vi "Teleop.vi"(10 "Match Info":T2={"Autonomous Elapsed Seconds"=0.0, "TeleOp Elapsed Seconds"=0.0, "Disabled Elapsed Seconds"=0.0, "Visited Autonomous"=FALSE, "Visited TeleOp"=FALSE, "Visited Disabled"=FALSE, "Autonomous Settings"={"Autonomous Style"=enum."Independent", "VI Refnum"=refnum}}, 11 "Call Context":T3) -> ()   [LabVIEW 2015]
doc: "This VI is called for each TeleOp packet received from the DS where the robot is not disabled. It is often used to read from the joysticks and update I/O or to update setpoints for timed control loops. It should complete and return within 20 milliseconds or it may miss DS packets."
uses:
  <vilib>/Rock Robotics/WPI/DriverStation/WPI_DriverStationDerivedRobotMode.ctl
  <vilib>/Rock Robotics/WPI/DriverStation/WPI_DriverStationMatch Info.ctl
  <vilib>/Rock Robotics/WPI/Utilities/WPI_GetSetVariantRefNum.vi
  <vilib>/Rock Robotics/Network Tables/SD Write Boolean Array.vi
  <vilib>/Rock Robotics/Network Tables/SD Read Boolean.vi
  <vilib>/Rock Robotics/Network Tables/SD Read Number.vi
  Robot Global Data.vi
  <vilib>/addons/control/pid/pid.llb/PID (DBL).vi
  <vilib>/Rock Robotics/WPI/RobotDrive/WPI_RobotDriveMecanumDrive_Cartesian.vi
  <vilib>/addons/control/pid/NI_PID_pid.lvlib
panel:
  in  "UseGyro?":bool
  out "Gyro":T1(graph)
  out "Rotation Input":dbl(graph)
  out "Sample Slider 0":dbl(slide) scale=0.0..5.0
  out "Sample Boolean 1":bool
  out "Sample Boolean 0":bool
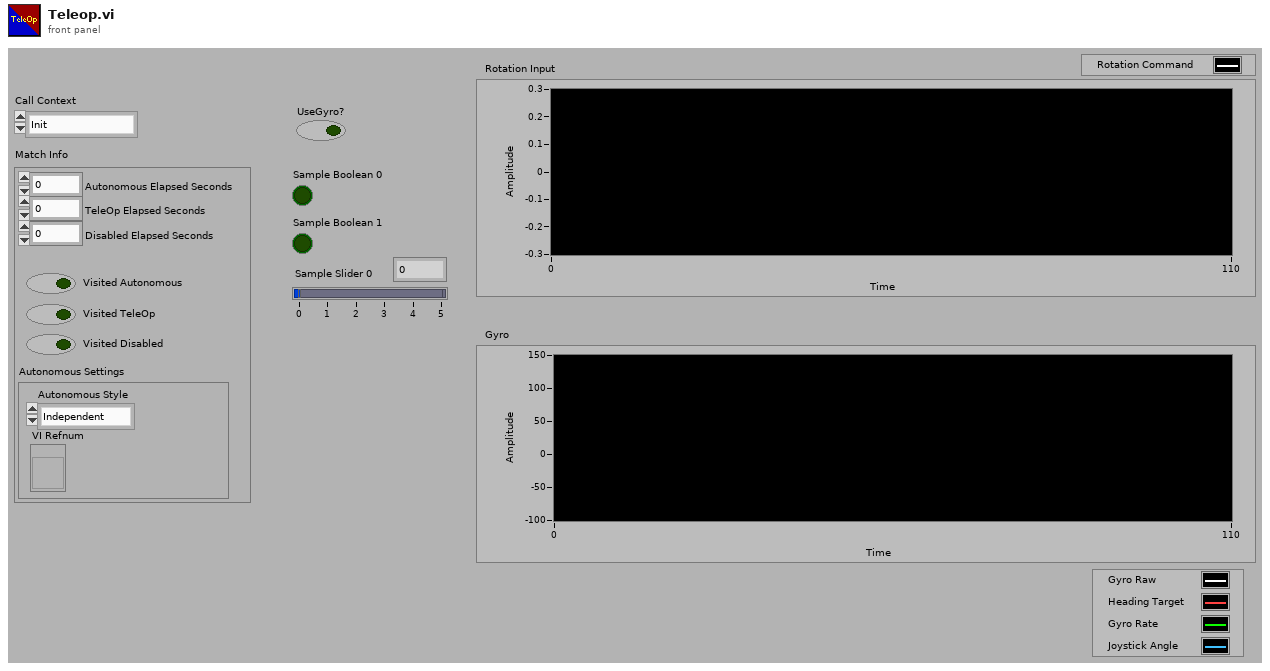
[diagram p1: front panel]
types:
  T1 = cluster{"Angle":dbl, "Heading":dbl, "Angular Rate":dbl, dbl}
  T2 = typedef "WPI_DriverStationMatch Info.ctl" = cluster{"Autonomous Elapsed Seconds":dbl, "TeleOp Elapsed Seconds":dbl, "Disabled Elapsed Seconds":dbl, "Visited Autonomous":bool, "Visited TeleOp":bool, "Visited Disabled":bool, "Autonomous Settings":cluster{"Autonomous Style":enum16{"Iterative", "Independent"}, "VI Refnum":refnum<vi>}}
  T3 = typedef "WPI_DriverStationDerivedRobotMode.ctl" = enum16{"Init", "Execute", "Stop"}
  T4 = cluster{"proportional gain (Kc)":dbl, "integral time (Ti, min)":dbl, "derivative time (Td, min)":dbl}
  T5 = typedef "WPI_JoystickDevRef.ctl" = cluster{"Device":T6}
  T6 = typedef "WPI_JoystickDeviceEnum.ctl" = enum16{"USB 0", "USB 1", "USB 2", "USB 3", "USB 4", "USB 5"}
  T7 = cluster{"Axes[0]":dbl, "Axes[1]":dbl, "Axes[2]":dbl, "Axes[3]":dbl, "Axes[4]":dbl, "Axes[5]":dbl, "Axes[6]":dbl, "Axes[7]":dbl, "Axes[8]":dbl}
  T8 = cluster{"Buttons[0]":bool, "Buttons[1]":bool, "Buttons[2]":bool, "Buttons[3]":bool, "Buttons[4]":bool, "Buttons[5]":bool, "Buttons[6]":bool, "Buttons[7]":bool, "Buttons[8]":bool}
  T9 = enum16{"CW_Fast", "CW_Slow", "CCW_Fast", "CCW_Slow", "Straight", "WaitingForStraight", "Rotate_Move"}
  T10 = cluster{"GyroHeading":dbl, "Heading":dbl, "GyroRate":dbl, dbl}
  T11 = typedef "WPI_RobotDriveDevRef.ctl" = cluster{"DevStatus":errorcluster, "Motors[]":T12[], "Square Inputs":bool, "Max Output":dbl}
  T12 = typedef "WPI_MotorControlDeviceRef.ctl" = cluster{"DeviceStatus":errorcluster, "Type":T13, "PWM":cluster{"PWM Channel":T14, "DeadBand":T15}, "CAN":cluster{"Device Number":u8, "Control Mode":T16, "Semaphore":T17, "Max Vout":dbl, "TalonSRX Control Mode":T18}, "Invert":bool}
  T13 = typedef "WPI_MotorControlType.ctl" = enum16{"PWM", "CAN", "CANTalonSRX"}
  T14 = typedef "FPGA_DIOPWMChannel.ctl" = enum8{"PWM 0", "PWM 1", "PWM 2", "PWM 3", "PWM 4", "PWM 5", "PWM 6", "PWM 7", "PWM 8", "PWM 9", "PWM MXP 0", "PWM MXP 1", "PWM MXP 2", "PWM MXP 3", "PWM MXP 4", "PWM MXP 5", "PWM MXP 6", "PWM MXP 7", "PWM MXP 8", "PWM MXP 9", "Invalid"}
  T15 = typedef "WPI_PWMDeadband.ctl" = cluster{"Name":string, "maxPositivePwm":i32, "minPositivePwm":i32, "centerPwm":i32, "maxNegativePwm":i32, "minNegativePwm":i32, "angularRange":u16}
  T16 = typedef "WPI_CANJaguar_ControlMode.ctl" = enum8{"Percent VBus", "Current", "Speed", "Position", "Voltage"}
  T17 = typedef "Semaphore RefNum" = refnum<k1>
  T18 = typedef "WPI_CANTalonSRX_APIControlMode.ctl" = enum8{"Percent VBus", "Speed", "Position", "Slave", "Unchanged / Invalid", "Voltage Compensation", "Current"}
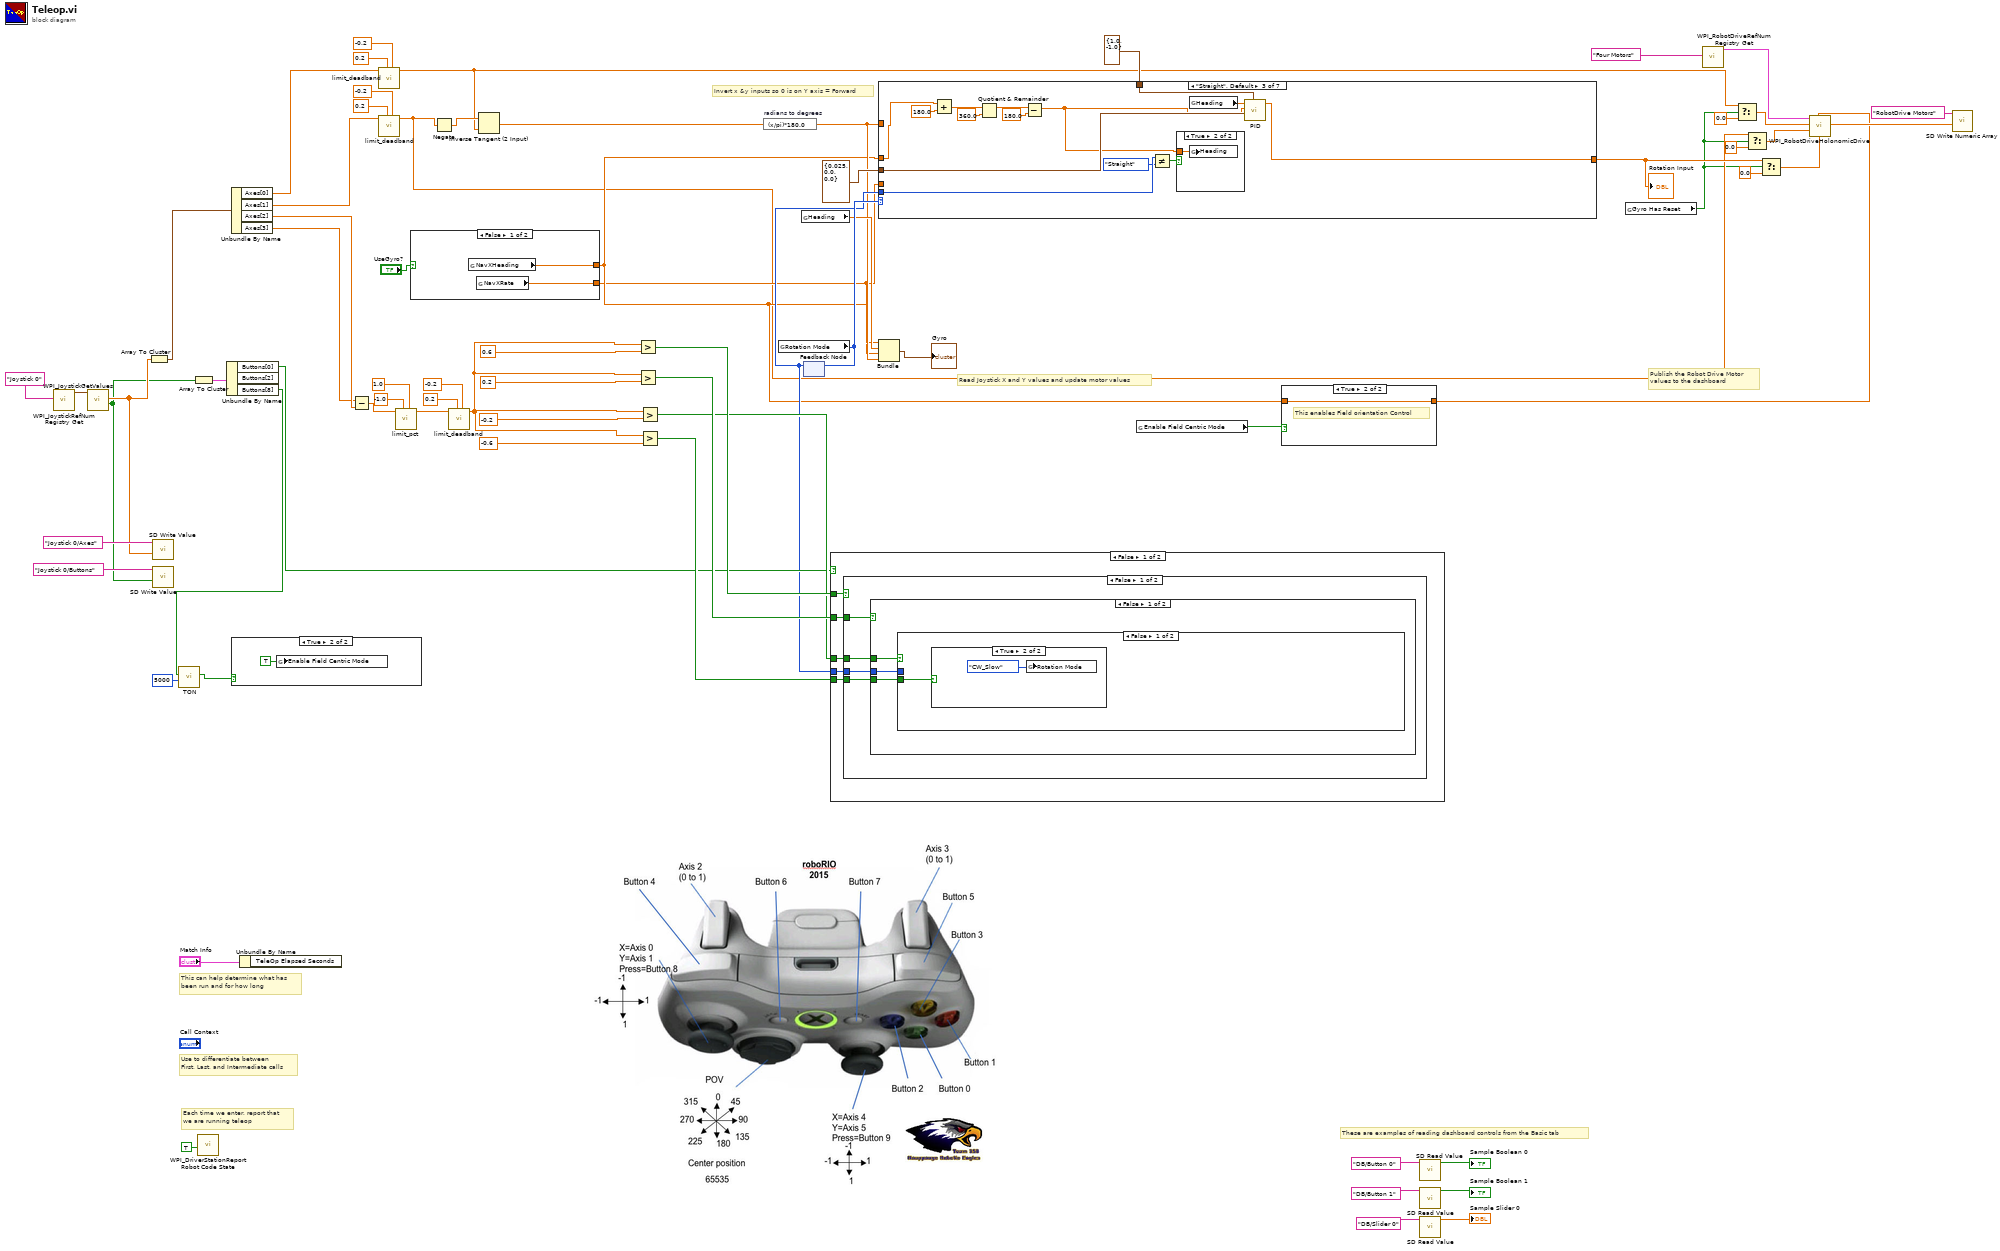
[diagram p0: block diagram]
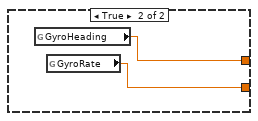
[diagram p2: hidden frame]
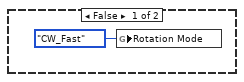
[diagram p4: hidden frame]
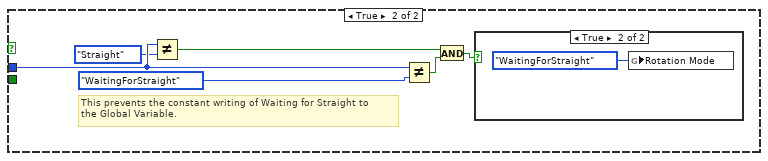
[diagram p5: hidden frame]
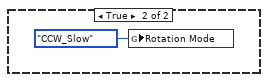
[diagram p7: hidden frame]
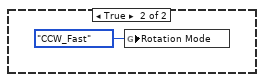
[diagram p8: hidden frame]
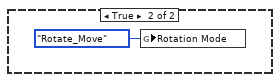
[diagram p9: hidden frame]
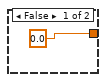
[diagram p10: hidden frame]
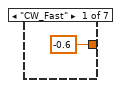
[diagram p11: hidden frame]
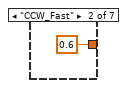
[diagram p12: hidden frame]
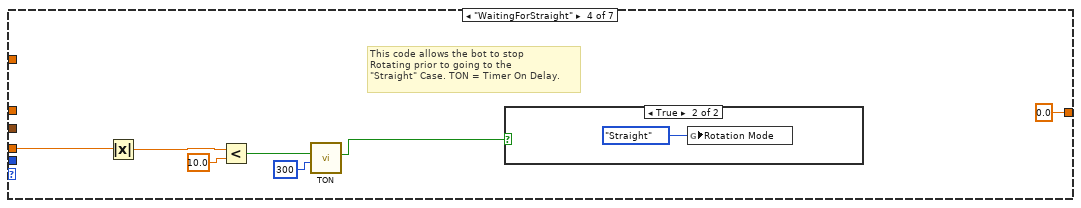
[diagram p14: hidden frame]
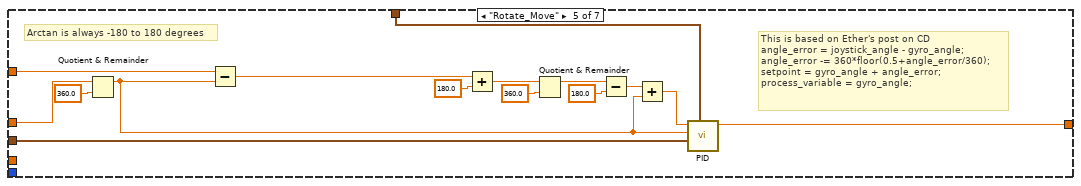
[diagram p16: hidden frame]
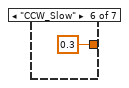
[diagram p17: hidden frame]
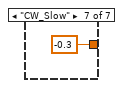
[diagram p18: hidden frame]
diagram:
  # "Invert x &y inputs so 0 is on Y axis = Forward"
  # "Publish the Robot Drive Motor\nvalues to the dashboard"
  # "Read Joystick X and Y values and update motor values"
  # "These are examples of reading dashboard controls from the Basic tab"
  # "Each time we enter, report that\nwe are running teleop"
  # "Use to differentiate between\nFirst, Last, and Intermediate calls"
  # "This can help determine what has\nbeen run and for how long"
  n1 = call <vilib>:"WPI_JoystickRefNum Registry Get.vi"("refnum name"="Joystick 0") -> ("JoystickDevRef"=w69:T5)  [unwired: 1 in, 9 out]
  n2 = call <vilib>:"WPI_JoystickGetValues.vi"("JoystickDevRef"=w69) -> ("Buttons"=w18:bool[], "Axes"=w20:dbl[])  [unwired: 6 in, 3 out]
  n3 = Array To Cluster(array=w20) -> (cluster=w19:T7)
  n4 = call-poly <vilib>:"SD Write Value.vi"("Numeric Array"=w20, "Name"="Joystick 0/Axes") -> ()  [unwired: 8 in, 2 out]
  n5 = call-poly <vilib>:"SD Write Value.vi"("Boolean Array"=w18, "Name"="Joystick 0/Buttons") -> ()  [unwired: 8 in, 2 out]
  n6 = Array To Cluster(array=w18) -> (cluster=w17:T8)
  n7 = call <vilib>:"WPI_DriverStationReport Robot Code State.vi"("TeleOp"=TRUE ("Autonomous")) -> ()  [unwired: 10 in, 1 out]
  n8 = Unbundle By Name(w17) -> ("Buttons[0]"=w36:bool, "Buttons[8]"=w12:bool)  [unwired: 1 out]
  n9 = call "TON.vi"("Delay (ms)"=u32 5000, "Input"=w12) -> ("Output"=w13:bool)  [unwired: 9 in]
  n10 = Unbundle By Name(w19) -> ("Axes[0]"=w35:dbl, "Axes[1]"=w24:dbl, "Axes[2]"=w27:dbl, "Axes[3]"=w26:dbl)
  n11 = case shown="True" w13 {
    frame False {
    }
    frame True {
      n12 = global write "Robot Global Data.vi" "Enable Field Centric Mode"(TRUE ("Enable Field Centric Mode")) -> ()
    }
  }
  n13 = Unbundle By Name("Match Info") -> ()  [unwired: 1 out]
  n14 = Subtract(x=w26, y=w27) -> (x-y=w28:dbl)
  n15 = call "limit_deadband.vi"("lower limit"=-0.2, "upper limit"=0.2, "Val"=w35) -> ("Val Out"=w3:dbl)  [unwired: 8 in]
  n16 = call "limit_deadband.vi"("lower limit"=-0.2, "upper limit"=0.2, "Val"=w24) -> ("Val Out"=w5:dbl)  [unwired: 8 in]
  n17 = call "limit_pct.vi"("upper limit"=1.0, "lower limit"=-1.0, "PCT"=w28) -> ("PCT Out"=w47:dbl)  [unwired: 8 in]
  n18 = case shown="False" "UseGyro?" {
    tunnel: [w74 w76] -> w15
    tunnel: [w73 w75] -> w14
    frame False {
      n19 = global read "Robot Global Data.vi" "NavXHeading"() -> (w74:dbl)
      n20 = global read "Robot Global Data.vi" "NavXRate"() -> (w73:dbl)
    }
    frame True {
      n21 = global read "Robot Global Data.vi" "GyroHeading"() -> (w76:dbl)
      n22 = global read "Robot Global Data.vi" "GyroRate"() -> (w75:dbl)
    }
  }
  n23 = Negate(x=w5) -> (-x=w23:dbl)
  n24 = call "limit_deadband.vi"("lower limit"=-0.2, "upper limit"=0.2, "Val"=w47) -> ("Val Out"=w40:dbl)  [unwired: 8 in]
  n25 = Inverse Tangent (2 Input)(1:w3, 2:w23) -> (0:w21:dbl)
  n26 = Greater?(x=w40, y=0.6 ("x")) -> (0:w46:bool)
  n27 = Greater?(x=w40, y=0.2 ("x")) -> (0:w45:bool)
  n28 = Greater?(x=w40, y=-0.2) -> (0:w41:bool)
  n29 = Greater?(x=w40, y=-0.6) -> (0:w38:bool)
  n30 = expression code="(x/pi)*180.0" "radians to degrees"(w21) -> (w22:dbl)
  n31 = global read "Robot Global Data.vi" "Rotation Mode"() -> (w32:T9)
  n32 = global read "Robot Global Data.vi" "Heading"() -> (w31:dbl)
  n33 = feedback #1() -> (w30:T9)  [unwired: 1 in]
  n34 = feedback-in #1(w32) -> ()
  n35 = case shown="False" w36 {
    tunnel: w46 -> [w81 _]
    tunnel: w45 -> [w80 _]
    tunnel: w41 -> [w79 _]
    tunnel: w38 -> [w78 _]
    tunnel: w30 -> [w77 _]
    frame False {
      n36 = case shown="False" w81 {
        tunnel: w80 -> [w85 _]
        tunnel: w79 -> [w84 _]
        tunnel: w78 -> [w83 _]
        tunnel: w77 -> [w82 _]
        frame False {
          n37 = case shown="False" w85 {
            tunnel: w84 -> [w88 _]
            tunnel: w83 -> [w87 _]
            tunnel: w82 -> [w86 _]
            frame False {
              n38 = case shown="False" w88 {
                tunnel: w87 -> [w89 _]
                tunnel: w86 -> [_ w97]
                frame False {
                  n39 = case shown="True" w89 {
                    frame False {
                      n40 = global write "Robot Global Data.vi" "Rotation Mode"(T9."CW_Fast" ("Rotation Mode")) -> ()
                    }
                    frame True {
                      n41 = global write "Robot Global Data.vi" "Rotation Mode"(T9."CW_Slow" ("Rotation Mode")) -> ()
                    }
                  }
                }
                frame True {
                  # "This prevents the constant writing of Waiting for Straight to \nthe Global Variable."
                  n42 = Not Equal?(x=w97, y=T9."Straight") -> (x != y?=w93:bool)
                  n43 = Not Equal?(x=w97, y=T9."WaitingForStraight") -> (x != y?=w92:bool)
                  n44 = And(x=w93, y=w92) -> (x .and. y?=w94:bool)
                  n45 = case shown="True" w94 {
                    frame False {
                    }
                    frame True {
                      n46 = global write "Robot Global Data.vi" "Rotation Mode"(T9."WaitingForStraight" ("Rotation Mode")) -> ()
                    }
                  }
                }
              }
            }
            frame True {
              n47 = global write "Robot Global Data.vi" "Rotation Mode"(T9."CCW_Slow" ("Rotation Mode")) -> ()
            }
          }
        }
        frame True {
          n48 = global write "Robot Global Data.vi" "Rotation Mode"(T9."CCW_Fast" ("Rotation Mode")) -> ()
        }
      }
    }
    frame True {
      n49 = global write "Robot Global Data.vi" "Rotation Mode"(T9."Rotate_Move" ("Rotation Mode")) -> ()
    }
  }
  n50 = case shown="\"Straight\", Default" w32 {
    tunnel: [-0.6 ("Rotation") 0.6 ("Rotation") w111 0.0 ("Rotation") w141 0.3 ("Rotation") -0.3 ("Rotation")] -> w9
    tunnel: w15 -> [_ _ w105 _ w128 _ _]
    tunnel: w14 -> [_ _ _ w120 _ _ _]
    tunnel: T4 {"proportional gain (Kc)"=0.025, "integral time (Ti, min)"=0.0, "derivative time (Td, min)"=0.0} ("PID gains") -> [_ _ w112 _ w140 _ _]
    tunnel: w22 -> [_ _ _ _ w134 _ _]
    tunnel: cluster{"output high":dbl, "output low":dbl} {"output high"=1.0, "output low"=-1.0} ("output range") -> [_ _ w113 _ w137 _ _]
    tunnel: w30 -> [_ _ w117 _ _ _ _]
    frame "CW_Fast" {
    }
    frame "CCW_Fast" {
    }
    frame "Straight", Default {
      n51 = Add(x=w105, y=180.0) -> (x+y=w108:dbl)
      n52 = Quotient & Remainder(x=w108, y=360.0) -> (x-y*floor(x/y)=w107:dbl)  [unwired: 1 out]
      n53 = Subtract(x=w107, y=180.0) -> (x-y=w104:dbl)
      n54 = Not Equal?(x=w117, y=T9."Straight" ("Rotation Mode")) -> (x != y?=w114:bool)
      n55 = case shown="True" w114 {
        tunnel: w104 -> [_ w118]
        frame False {
        }
        frame True {
          n56 = global write "Robot Global Data.vi" "Heading"(w118) -> ()
        }
      }
      n57 = global read "Robot Global Data.vi" "Heading"() -> (w115:dbl)
      n58 = call-poly <vilib>:"PID.vi"("output range"=w113, "PID gains"=w112, "process variable"=w104, "setpoint"=w115) -> ("output"=w111:dbl)  [unwired: 6 in, 1 out]
    }
    frame "WaitingForStraight" {
      # "This code allows the bot to stop \nRotating prior to going to the \n\"Straight\" Case. TON = Timer On Delay."
      n59 = Absolute Value(x=w120) -> (abs(x)=w119:dbl)
      n60 = Less?(x=w119, y=10.0) -> (x < y?=w122:bool)
      n61 = call "TON.vi"("Delay (ms)"=u32 300, "Input"=w122) -> ("Output"=w123:bool)  [unwired: 9 in]
      n62 = case shown="True" w123 {
        frame False {
        }
        frame True {
          n63 = global write "Robot Global Data.vi" "Rotation Mode"(T9."Straight" ("Rotation Mode")) -> ()
        }
      }
    }
    frame "Rotate_Move" {
      # "Arctan is always -180 to 180 degrees"
      # "This is based on Ether's post on CD\nangle_error = joystick_angle - gyro_angle;\nangle_error -= 360*floor(0.5+angle_error/360);\nsetpoint = gyro_angle + angle_error;\nprocess_variable = gyro_angle;"
      n64 = Quotient & Remainder(x=w128, y=360.0) -> (x-y*floor(x/y)=w127:dbl)  [unwired: 1 out]
      n65 = Subtract(x=w134, y=w127) -> (x-y=w136:dbl)
      n66 = Add(x=w136, y=180.0) -> (x+y=w133:dbl)
      n67 = Quotient & Remainder(x=w133, y=360.0) -> (x-y*floor(x/y)=w132:dbl)  [unwired: 1 out]
      n68 = Subtract(x=w132, y=180.0) -> (x-y=w130:dbl)
      n69 = Add(x=w130, y=w127) -> (x+y=w129:dbl)
      n70 = call-poly <vilib>:"PID.vi"("output range"=w137, "PID gains"=w140, "process variable"=w127, "setpoint"=w129) -> ("output"=w141:dbl)  [unwired: 6 in, 1 out]
    }
    frame "CCW_Slow" {
    }
    frame "CW_Slow" {
    }
  }
  "Rotation Input" <- w9
  n71 = Bundle("GyroHeading"=w15, "Heading"=w31, "GyroRate"=w14, w22) -> (→"Gyro":T10)  [unwired: 1 in]
  n72 = global read "Robot Global Data.vi" "Enable Field Centric Mode"() -> (w25:bool)
  n73 = case shown="True" w25 {
    tunnel: w15 -> [_ w145]
    tunnel: [0.0 ("Angle") w145] -> w37
    frame False {
    }
    frame True {
      # "This enables Field orientation Control"
    }
  }
  n74 = call-poly <vilib>:"SD Read Value.vi"("Name"="DB/Button 0" ("refnum name")) -> ("Boolean"=→"Sample Boolean 0":bool)  [unwired: 8 in, 2 out]
  n75 = call-poly <vilib>:"SD Read Value.vi"("Name"="DB/Button 1" ("refnum name")) -> ("Boolean"=→"Sample Boolean 1":bool)  [unwired: 8 in, 2 out]
  n76 = call-poly <vilib>:"SD Read Value.vi"("Name"="DB/Slider 0" ("refnum name")) -> ("Numeric"=→"Sample Slider 0":dbl)  [unwired: 8 in, 2 out]
  n77 = global read "Robot Global Data.vi" "Gyro Has Reset"() -> (w1:bool)
  n78 = call <vilib>:"WPI_RobotDriveRefNum Registry Get.vi"("refnum name"="Four Motors") -> ("RobotDriveDevRef"=w58:T11)  [unwired: 1 in, 9 out]
  n79 = Select(t=w3, s=w1, f=0.0) -> (s? t:f=w2:dbl)
  n80 = Select(t=w5, s=w1, f=0.0) -> (s? t:f=w6:dbl)
  n81 = Select(t=w9, s=w1, f=0.0) -> (s? t:f=w10:dbl)
  n82 = call-poly <vilib>:"WPI_RobotDriveHolonomicDrive.vi"("Rotation"=w10, "Gyro Angle"=w37, "Y"=w6, "X"=w2, "RobotDriveDevRef"=w58) -> ("Motor Values"=w56:dbl[])  [unwired: 4 in, 2 out]
  n83 = call <vilib>:"SD Write Numeric Array.vi"("Numeric Array"=w56, "Name"="RobotDrive Motors") -> ()  [unwired: 8 in, 2 out]
